vi "Lab1.vi"() -> ()   [LabVIEW 2015]
panel:
  out "Array 4":string[](array[string])
  in  "Array 3":string[](array[string])
  out "Path 2":path
  in  "Path":path
  out "Boolean 2":bool
  in  "Boolean":bool
  out "String 3":string
  out "String 2":string
  in  "String":string
  out "Numeric 3":dbl
  in  "Numeric 2":dbl
  out "Numeric":i32
  out "Array 2":dbl[](array[numeric])
  in  "Array":dbl[](array[numeric])
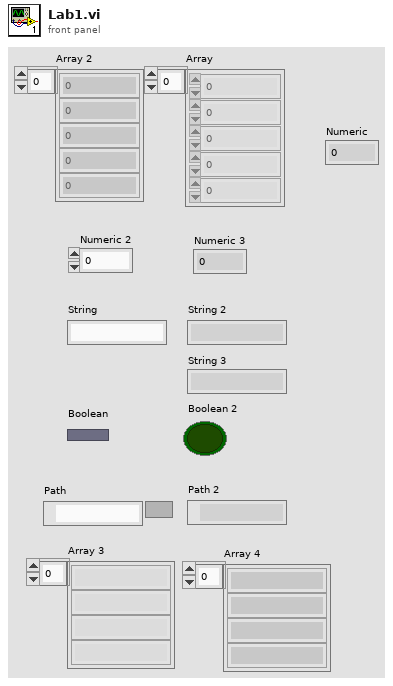
[diagram p1: front panel]
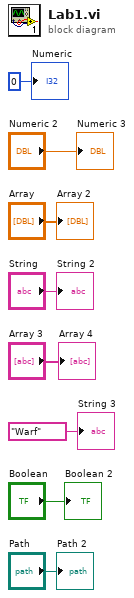
[diagram p0: block diagram]
diagram:
  "Array 2" <- "Array"
  "Numeric" <- 0
  "Numeric 3" <- "Numeric 2"
  "String 2" <- "String"
  "String 3" <- "Warf"
  "Boolean 2" <- "Boolean"
  "Path 2" <- "Path"
  "Array 4" <- "Array 3"
